vi "Folder - Subtract Number of Months.vi"(9 "- # of Months":i32, 10 "YYYYmm":string, 11 "Folder":path=path "C:/Temp1") -> (1 "< Range (Folder\\YYYY\\mm)":path[](array[path]), 2 ">= Range (Folder\\YYYY\\mm)":path[](array[path]), 3 "Folder\\YYYY\\mm":path[](array[path]))   [LabVIEW 2013]
panel:
  out "YYYYmm":i32[](array[numeric])
  out "YYYYmm - # of Months":i32
  out "YYYYmm":string[](array[string])
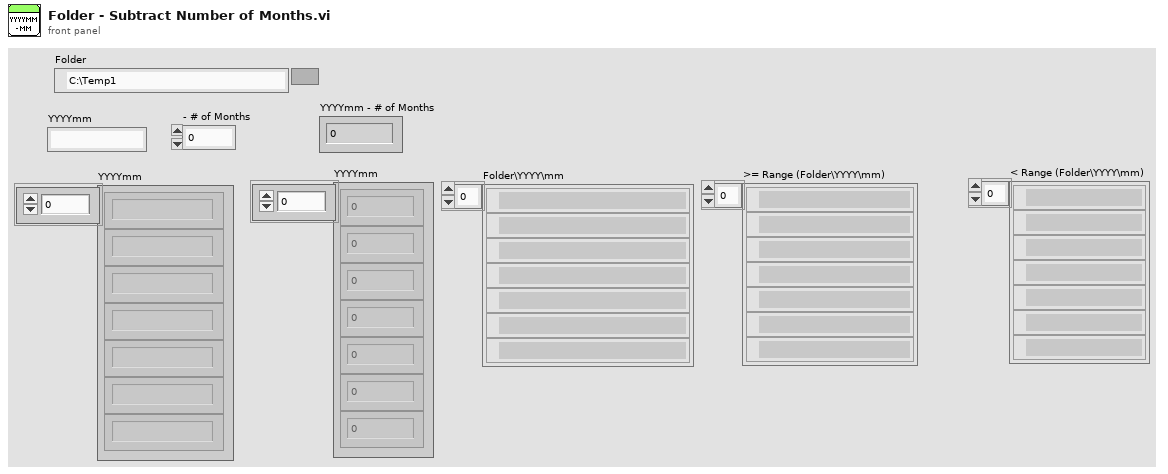
[diagram p1: front panel]
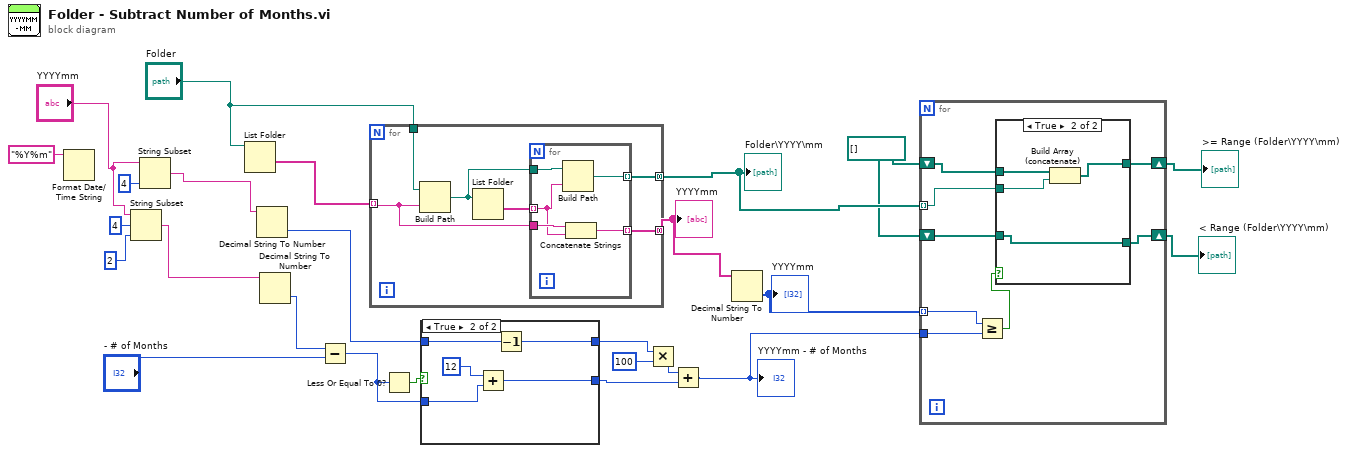
[diagram p0: block diagram]
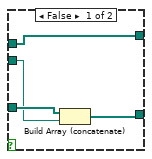
[diagram p2: hidden frame]
diagram:
  w1 = path[] []
  n1 = Format Date/Time String(time format string (%c)="%Y%m") -> ()  [unwired: 2 in, 1 out]
  n2 = String Subset(string="YYYYmm", offset (0)=4, length (rest)=2 ("length (rest)")) -> (substring=w8:string)
  n3 = String Subset(string="YYYYmm", length (rest)=4 ("length (rest)")) -> (substring=w9:string)  [unwired: 1 in]
  n4 = List Folder(path="Folder") -> (folder names=w25:string[])  [unwired: 3 in, 3 out]
  n5 = Decimal String To Number(string=w9) -> (number=w20:i32)  [unwired: 2 in, 1 out]
  n6 = Decimal String To Number(string=w8) -> (number=w23:i32)  [unwired: 2 in, 1 out]
  n7 = Subtract(x=w23, y="- # of Months") -> (x-y=w19:i32)
  n8 = for {
    tunnel: w25 -> [w30] mode=indexing
    tunnel: "Folder" -> [w31]
    tunnel: [w29] -> w15 mode=concatenating
    tunnel: [w26] -> w4 mode=concatenating
    n9 = Build Path(base path=w31, name or relative path=w30) -> (appended path=w27:path)
    n10 = List Folder(path=w27) -> (folder names=w28:string[])  [unwired: 3 in, 3 out]
    n11 = for {
      tunnel: w30 -> [w36]
      tunnel: w28 -> [w33] mode=indexing
      tunnel: [w35] -> w29 mode=indexing
      tunnel: w27 -> [w34]
      tunnel: [w32] -> w26 mode=indexing
      n12 = Build Path(base path=w34, name or relative path=w33) -> (appended path=w32:path)
      n13 = Concatenate Strings(w36, w33) -> (w35:string)
    }
  }
  "YYYYmm" <- w15
  "Folder\\YYYY\\mm" <- w4
  n14 = Less Or Equal To 0?(x=w19) -> (x <= 0?=w21:bool)
  n15 = case shown="True" w21 {
    tunnel: w19 -> [w37 w42]
    tunnel: w20 -> [w38 w41]
    tunnel: [w37 w39] -> w14
    tunnel: [w38 w40] -> w16
    frame False {
    }
    frame True {
      n16 = Add(x=12, y=w42) -> (x+y=w39:i32)
      n17 = Decrement(x=w41) -> (x-1=w40:i32)
    }
  }
  n18 = Multiply(x=w16, y=100) -> (x*y=w18:i32)
  n19 = Add(x=w18, y=w14) -> (x+y=w5:i32)
  "YYYYmm - # of Months" <- w5
  n20 = Decimal String To Number(string=w15) -> (number=w6:i32[])  [unwired: 2 in, 1 out]
  "YYYYmm" <- w6
  n21 = for {
    tunnel: w6 -> [w51] mode=indexing
    tunnel: w5 -> [w50]
    tunnel: w4 -> [w49] mode=indexing
    shift-right: [w46] -> w3
    shift-left: w1 -> [w47]
    shift-right: [w44] -> w2
    shift-left: w1 -> [w45]
    n22 = Greater Or Equal?(x=w51, y=w50) -> (x >= y?=w48:bool)
    n23 = case shown="True" w48 {
      tunnel: w49 -> [w53 w57]
      tunnel: [w54 w56] -> w44
      tunnel: w47 -> [w52 w59]
      tunnel: [w52 w58] -> w46
      tunnel: w45 -> [w55 w56]
      frame False {
        n24 = Build Array (concatenate)(w55, w53) -> (w54:path[])
      }
      frame True {
        n25 = Build Array (concatenate)(w59, w57) -> (w58:path[])
      }
    }
  }
  ">= Range (Folder\\YYYY\\mm)" <- w3
  "< Range (Folder\\YYYY\\mm)" <- w2
